vi "Dense - Scale Nodes Linear.vi"(8 "error in (no error)":errorcluster, 9 "Scaling limits":cluster{"X lower":dbl, "X upper":dbl}, 10 "xmaxmin":cluster{"min":dbl, "max":dbl}[](array[cluster]), 11 "x":dbl[](array[numeric])) -> (0 "error out":errorcluster, 3 "x scaled":dbl[](array[numeric]))   [LabVIEW 2014]
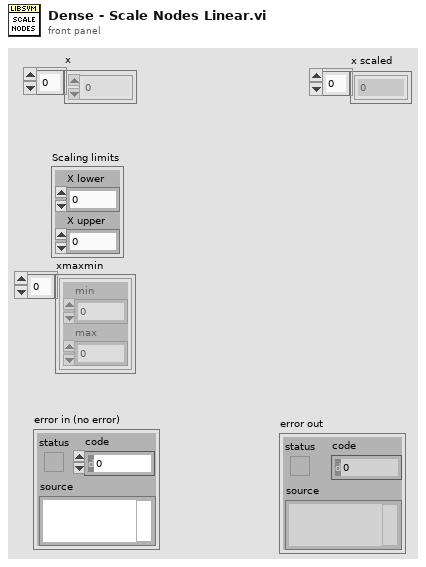
[diagram p1: front panel]
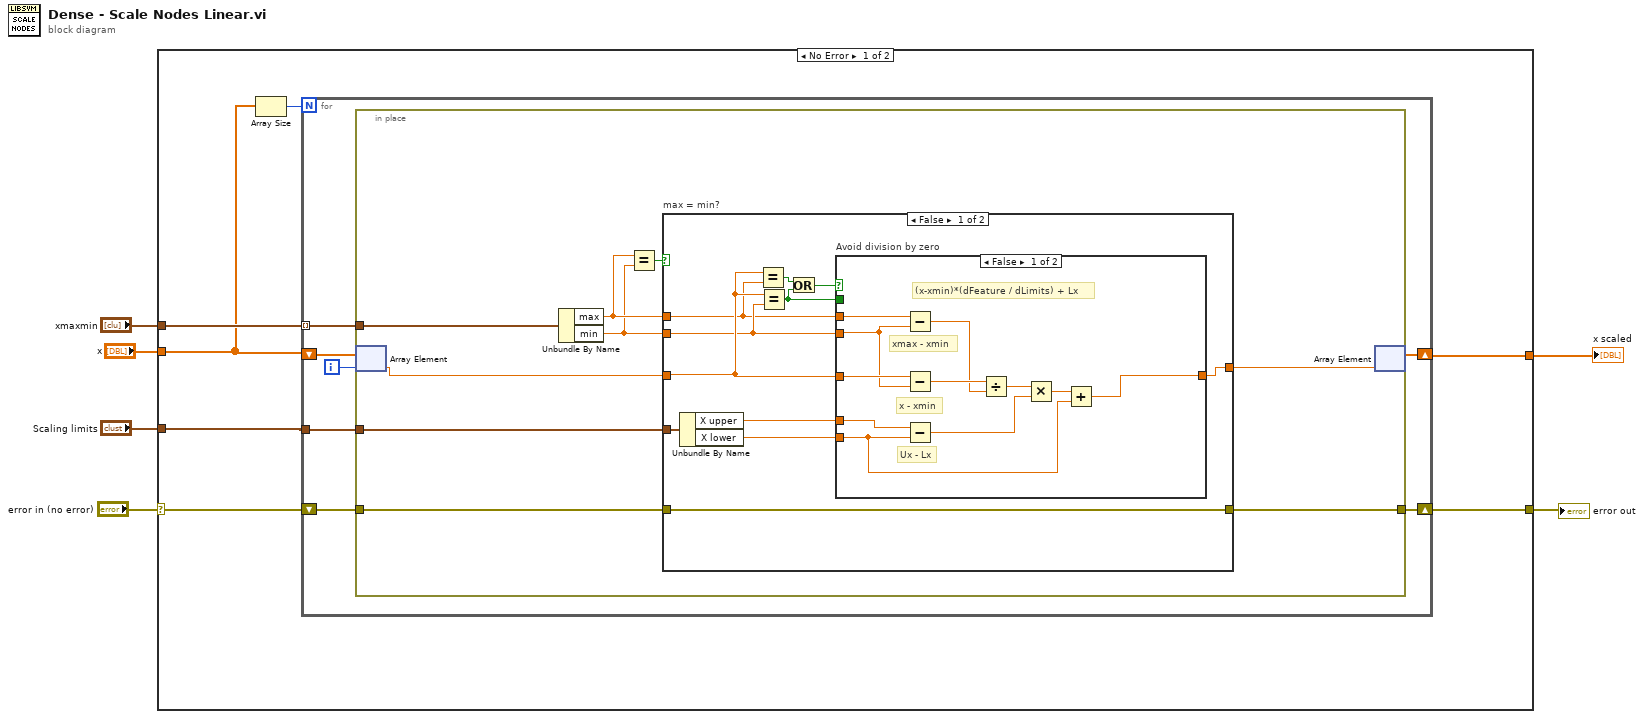
[diagram p0: block diagram]
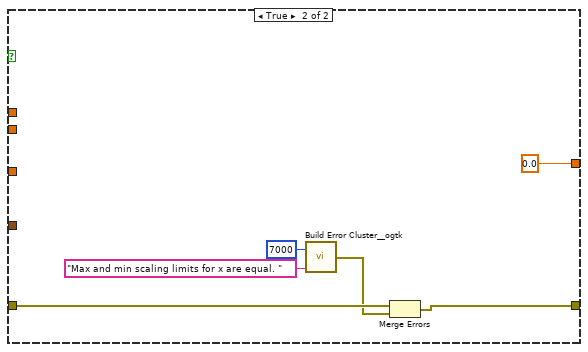
[diagram p4: hidden frame]
diagram:
  n1 = case shown="No Error" "error in (no error)" {
    selector: "error in (no error)" -> [w8 w64]
    tunnel: [w7 w64] -> w6
    tunnel: "Scaling limits" -> [w13 _]
    tunnel: "xmaxmin" -> [w12 _]
    tunnel: [w10 _] -> w1
    tunnel: "x" -> [w9 _]
    frame No Error {
      n2 = Array Size(array=w9) -> (size(s)=w11:i32)
      n3 = for {
        N: w11 -> [_]
        shift-right: [w19] -> w10
        shift-left: w9 -> [w20]
        tunnel: w12 -> [w18] mode=indexing
        tunnel: w13 -> [w17]
        shift-right: [w14] -> w7
        shift-left: w8 -> [w15]
        i -> [w16]
        n4 = in-place {
          in-place-border: w18 -> [w25]
          in-place-border: w17 -> [w29]
          in-place-border: w15 -> [w22]
          in-place-border: [w21] -> w14
          n5 = in-place-array #1(w20, w16) -> (w24:dbl)
          n6 = Unbundle By Name(w25) -> ("max"=w27:dbl, "min"=w26:dbl)
          n7 = Equal?(x=w27, y=w26) -> (x = y?=w28:bool)
          n8 = case "max = min?" shown="False" w28 {
            tunnel: w27 -> [w35 _]
            tunnel: w26 -> [w36 _]
            tunnel: w24 -> [w37 _]
            tunnel: w29 -> [w40 _]
            tunnel: [w31 0.0 ("value")] -> w23
            tunnel: w22 -> [w30 w60]
            tunnel: [w30 w58] -> w21
            frame False {
              # "maxmin not equal"
              n9 = Unbundle By Name(w40) -> ("X upper"=w33:dbl, "X lower"=w32:dbl)
              n10 = Equal?(x=w37, y=w35) -> (x = y?=w39:bool)
              n11 = Equal?(x=w37, y=w36) -> (x = y?=w34:bool)
              n12 = Or(x=w39, y=w34) -> (x .or. y?=w38:bool)
              n13 = case "Avoid division by zero" shown="False" w38 {
                tunnel: w37 -> [w50 _]
                tunnel: w35 -> [w49 _]
                tunnel: w36 -> [w48 _]
                tunnel: w34 -> [_ w55]
                tunnel: w33 -> [w51 w54]
                tunnel: w32 -> [w42 w53]
                tunnel: [w41 w52] -> w31
                frame False {
                  # "(x-xmin)*(dFeature / dLimits) + Lx"
                  # "xmax - xmin"
                  # "x - xmin"
                  # "Ux - Lx"
                  n14 = Subtract(x=w49, y=w48) -> (x-y=w46:dbl)
                  n15 = Subtract(x=w50, y=w48) -> (x-y=w47:dbl)
                  n16 = Subtract(x=w51, y=w42) -> (x-y=w44:dbl)
                  n17 = Divide(x=w47, y=w46) -> (x/y=w45:dbl)
                  n18 = Multiply(x=w45, y=w44) -> (x*y=w43:dbl)
                  n19 = Add(x=w43, y=w42) -> (x+y=w41:dbl)
                }
                frame True {
                  n20 = case shown="True" w55 {
                    tunnel: w54 -> [w56 _]
                    tunnel: w53 -> [_ w57]
                    tunnel: [w56 w57] -> w52
                    frame False {
                    }
                    frame True {
                    }
                  }
                }
              }
            }
            frame True {
              # "set to"
              n21 = call <userlib>:"Build Error Cluster__ogtk.vi"("String to Prepend to source (\"\")"="Max and min scaling limits for x are equal. " ("String to Prepend to source (\"\")"), "code"=7000) -> ("error out"=w59:errorcluster)
              n22 = Merge Errors(w60, w59) -> (w58:errorcluster)
            }
          }
          n23 = in-place-array #1(w23) -> (w19:dbl[])  [unwired: 1 out]
        }
      }
    }
    frame Error {
    }
  }
  "error out" <- w6
  "x scaled" <- w1
